vi "CFTS-Get Acoustic System IDs.vi"(8 "error in (no error)":errorcluster) -> (0 "error out":errorcluster, 2 "Left":string, 3 "Right":string)   [LabVIEW 2020]
uses:
  <vilib>/Utility/config.llb/Read Key (String).vi
  <vilib>/Utility/config.llb/NI_LVConfig.lvlib
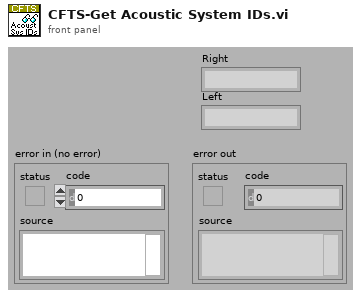
[diagram p1: front panel]
types:
  T1 = typedef "NI_LVConfig.lvlib/Config Data RefNum.ctl" = refnum<k1>
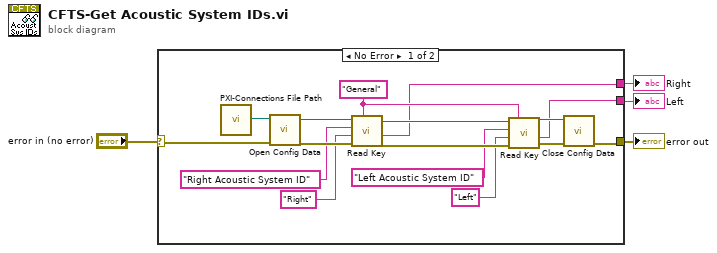
[diagram p0: block diagram]
diagram:
  n1 = case shown="No Error" "error in (no error)" {
    selector: "error in (no error)" -> [w20 w21]
    tunnel: [w10 w21] -> w4
    tunnel: [w7 _] -> w1
    tunnel: [w6 _] -> w2
    frame No Error {
      w15 = "General" ("section")
      n2 = call "PXI-Connections File Path.vi"() -> ("Path"=w5:path)  [unwired: 1 in]
      n3 = call <vilib>:"Open Config Data.vi"("error in (no error)"=w20, "configuration file path"=w5) -> ("error out"=w19:errorcluster, "refnum"=w18:T1)  [unwired: 7 in, 1 out]
      n4 = call-poly <vilib>:"Read Key.vi"("section"=w15, "error in (no error)"=w19, "default value"="Right" ("key"), "key"="Right Acoustic System ID", "refnum"=w18) -> ("error out"=w13:errorcluster, "value"=w6:string, "refnum out"=w14:T1)  [unwired: 3 in, 1 out]
      n5 = call-poly <vilib>:"Read Key.vi"("section"=w15, "error in (no error)"=w13, "default value"="Left" ("key"), "key"="Left Acoustic System ID", "refnum"=w14) -> ("error out"=w9:errorcluster, "value"=w7:string, "refnum out"=w8:T1)  [unwired: 3 in, 1 out]
      n6 = call <vilib>:"Close Config Data.vi"("error in (no error)"=w9, "refnum"=w8) -> ("error out"=w10:errorcluster)  [unwired: 8 in, 1 out]
    }
    frame Error {
    }
  }
  "error out" <- w4
  "Right" <- w2
  "Left" <- w1
